vi "Autonomous Independent.vi"() -> ()   [LabVIEW 2014]
doc: "This VI is called when autonomous begins, and will automatically be terminated when autonomous ends. You can carry out timed or sensor driven robot movement independently without needing to return to the caller."
uses:
  <vilib>/Rock Robotics/WPI/Joystick/WPI_JoystickGetSetRefNum.vi
  Global Variables.vi
panel:
  out "Elapsed Time (s)":dbl
  out "Case":i32
  out "Array":dbl[][](array[numeric])
  # "Be sure to right-click and choose Data Operations>>Make Current Value default if you want to save the array values with the VI"
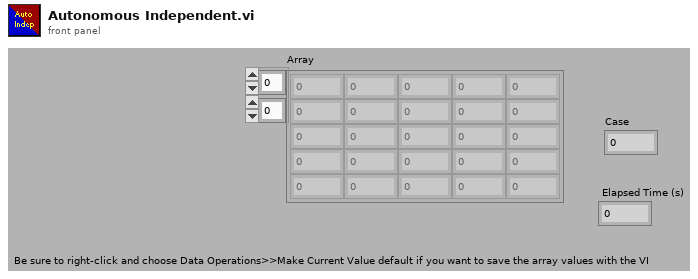
[diagram p1: front panel]
types:
  T1 = typedef "WPI_JoystickDevRef.ctl" = cluster{"Device":T2}
  T2 = typedef "WPI_JoystickDeviceEnum.ctl" = enum16{"USB 0", "USB 1", "USB 2", "USB 3", "USB 4", "USB 5"}
  T3 = typedef "WPI_CounterDevRef.ctl" = cluster{"DevStatus":errorcluster, "CntIndex":T4}
  T4 = typedef "FPGA_CounterCtrSystemIndex.ctl" = enum8{"Ctr 0", "Ctr 1", "Ctr 2", "Ctr 3", "Ctr 4", "Ctr 5", "Ctr 6", "Ctr 7", "Invalid"}
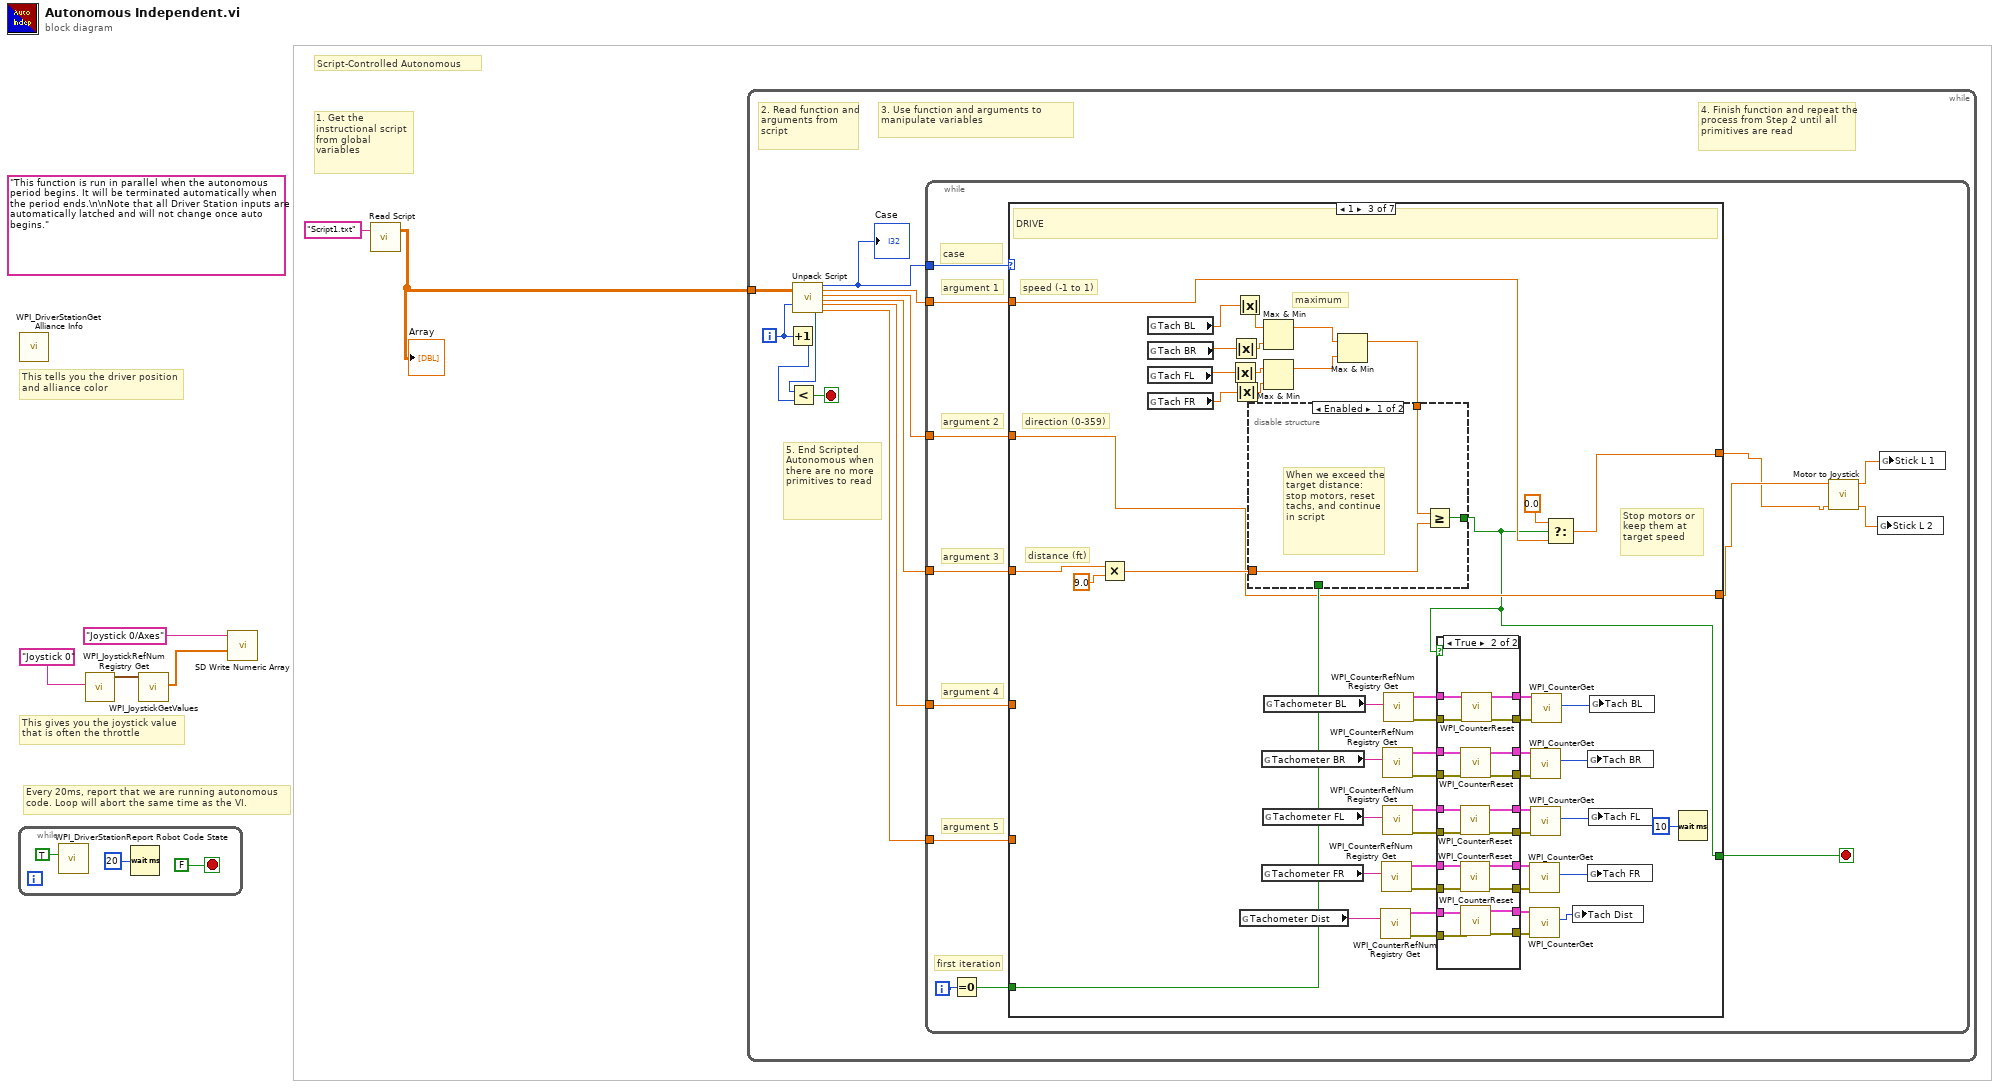
[diagram p0: block diagram]
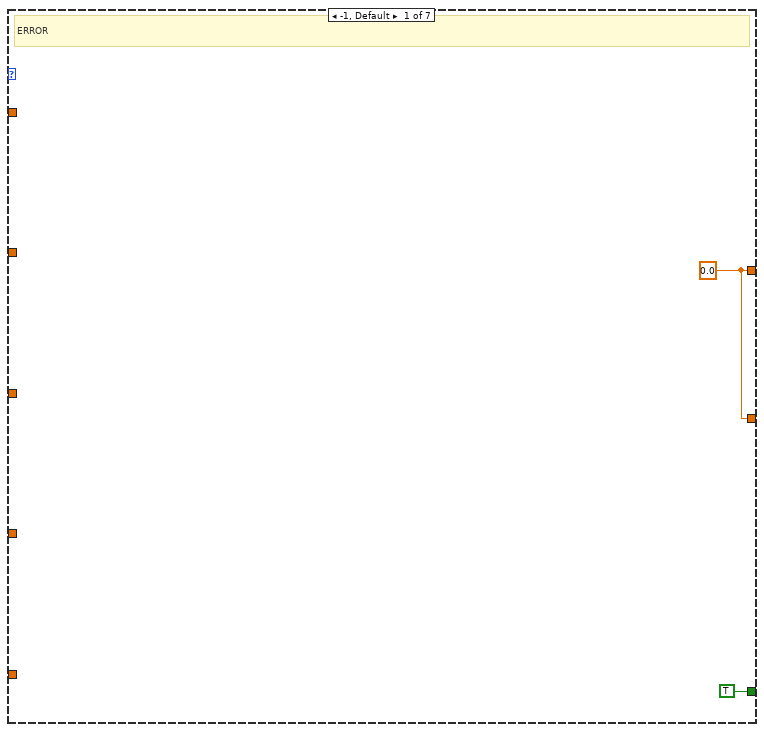
[diagram p2: hidden frame]
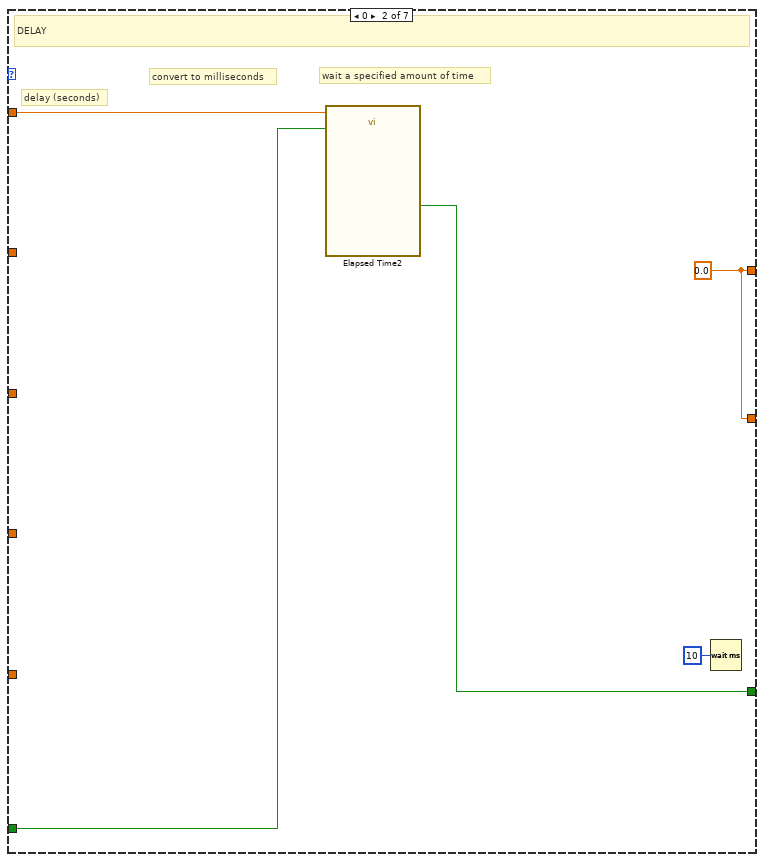
[diagram p3: hidden frame]
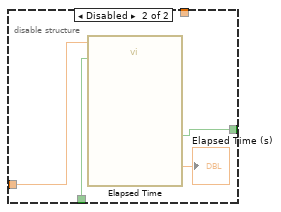
[diagram p5: hidden frame]
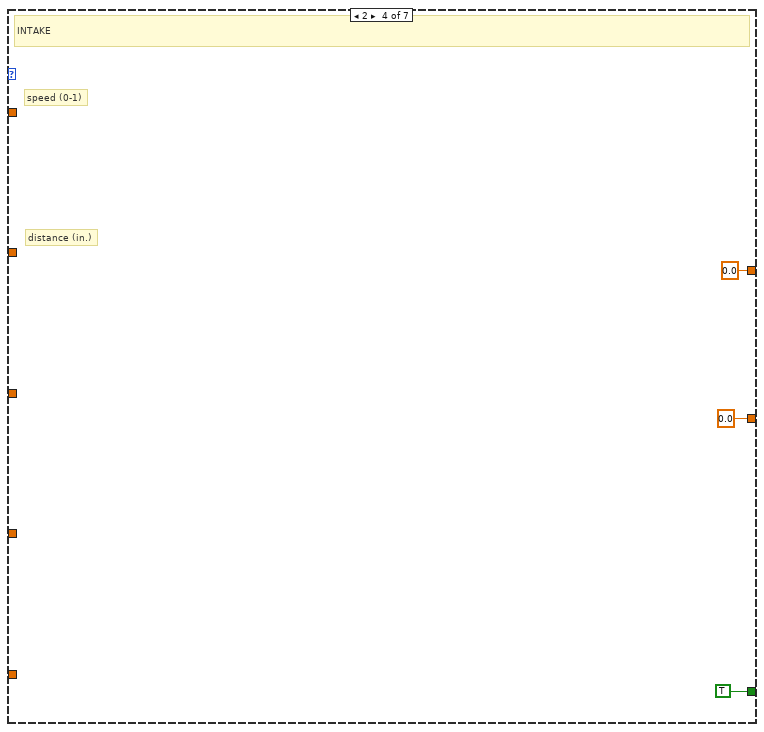
[diagram p6: hidden frame]
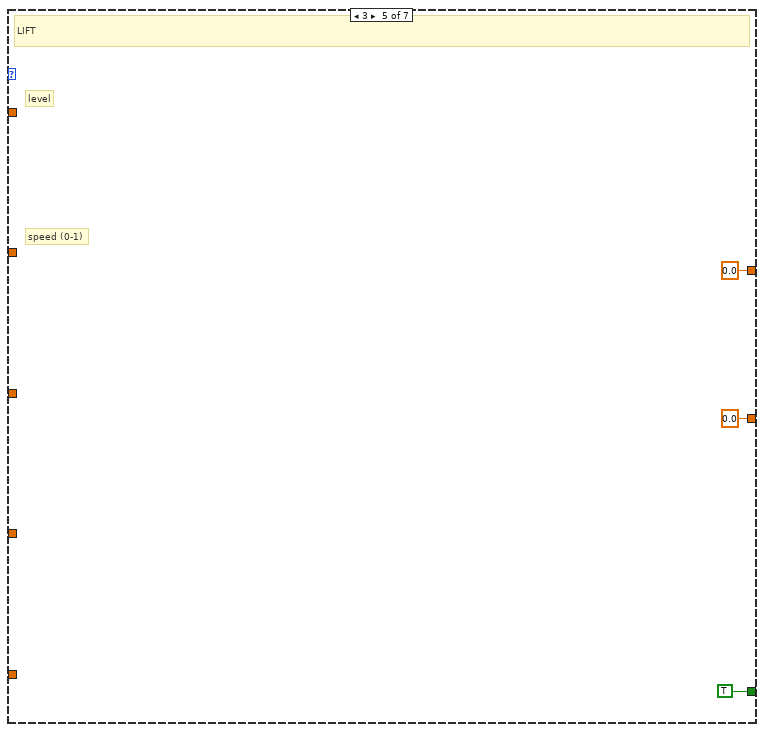
[diagram p7: hidden frame]
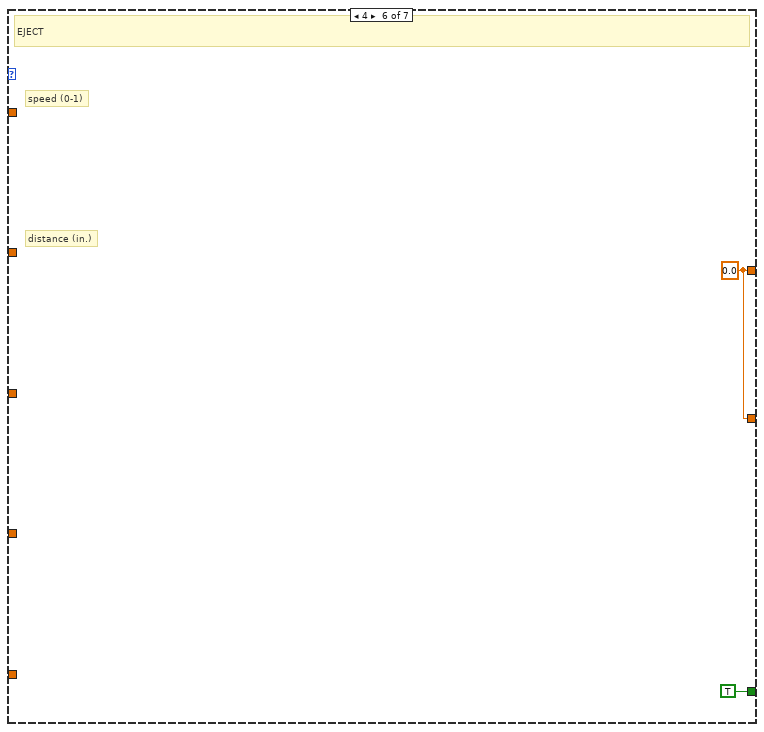
[diagram p8: hidden frame]
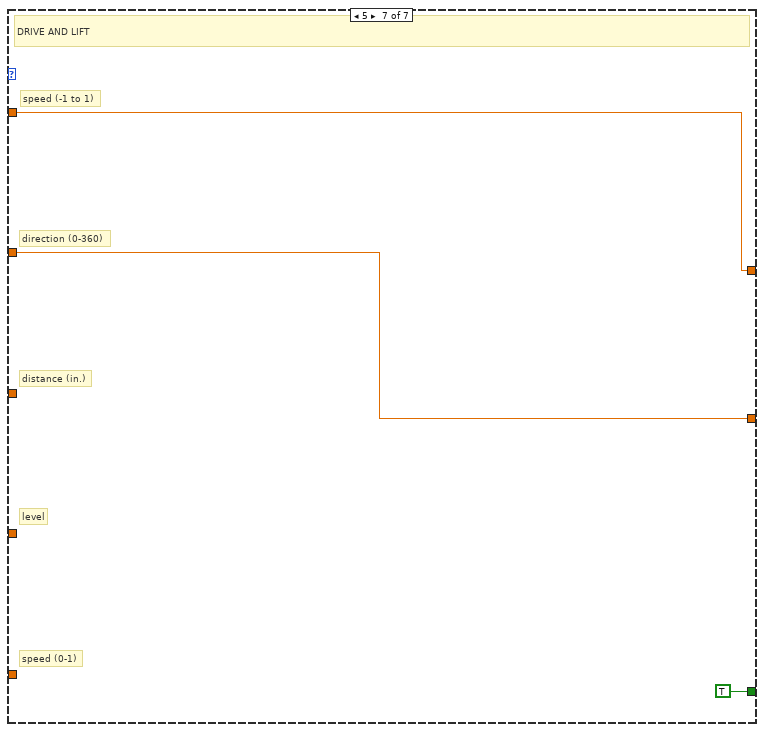
[diagram p9: hidden frame]
diagram:
  (unwired) "This function is run in parallel when the autonomous period begins. It will be terminated automatically when the period ends.\n\nNote that all Driver Station inputs are automatically latched and will not change once auto begins."
  # "1. Get the instructional script from global variables"
  # "Script-Controlled Autonomous"
  # "Every 20ms, report that we are running autonomous\ncode. Loop will abort the same time as the VI."
  # "This gives you the joystick value\nthat is often the throttle"
  # "This tells you the driver position\nand alliance color"
  n1 = while {
    stop <- FALSE stop-if-true
    n2 = call <vilib>:"WPI_DriverStationReport Robot Code State.vi"("Autonomous"=TRUE) -> ()  [unwired: 10 in, 1 out]
    n3 = Wait (ms)(milliseconds to wait=u32 20) -> ()  [unwired: 1 out]
  }
  n4 = call <vilib>:"WPI_DriverStationGet Alliance Info.vi"() -> ()  [unwired: 12 out]
  n5 = call <vilib>:"WPI_JoystickRefNum Registry Get.vi"("refnum name"="Joystick 0") -> ("JoystickDevRef"=w5:T1)  [unwired: 1 in, 9 out]
  n6 = call <vilib>:"WPI_JoystickGetValues.vi"("JoystickDevRef"=w5) -> ("Axes"=w3:dbl[])  [unwired: 6 in, 4 out]
  n7 = call <vilib>:"SD Write Numeric Array.vi"("Numeric Array"=w3, "Name"="Joystick 0/Axes") -> ()  [unwired: 8 in, 2 out]
  n8 = call "Read Script.vi"("script name"="Script1.txt") -> ("output array"=w1:dbl[][])  [unwired: 1 in, 1 out]
  "Array" <- w1
  n9 = while {
    tunnel: w1 -> [w11]
    i -> [w14]
    stop <- w20 stop-if-true
    # "4. Finish function and repeat the process from Step 2 until all primitives are read"
    # "3. Use function and arguments to manipulate variables"
    # "5. End Scripted Autonomous when there are no more primitives to read"
    # "2. Read function and arguments from script"
    n10 = Increment(x=w14) -> (x+1=w13:i32)
    n11 = call "Unpack Script.vi"("script"=w11, "index"=w14) -> ("# of primitives"=w12:i32, "primitive"=w10:i32, "argument 1"=w19:dbl, "argument 2"=w18:dbl, "argument 3"=w17:dbl, "argument 4"=w16:dbl, "argument 5"=w15:dbl)  [unwired: 11 in]
    "Case" <- w10
    n12 = Less?(x=w12, y=w13) -> (x < y?=w20:bool)
    n13 = while {
      tunnel: w19 -> [w33]
      tunnel: w18 -> [w32]
      tunnel: w17 -> [w31]
      tunnel: w16 -> [w30]
      tunnel: w15 -> [w29]
      tunnel: w10 -> [w28]
      i -> [w26]
      stop <- w27 stop-if-true
      # "first iteration"
      # "case"
      # "argument 5"
      # "argument 4"
      # "argument 3"
      # "argument 2"
      # "argument 1"
      n14 = Equal To 0?(x=w26) -> (x = 0?=w25:bool)
      n15 = case shown="1" w28 {
        tunnel: w33 -> [_ w40 w91 _ _ _ w138]
        tunnel: w32 -> [_ _ w80 _ _ _ w137]
        tunnel: w31 -> [_ _ w87 _ _ _ _]
        tunnel: w30 -> [_ _ _ _ _ _ _]
        tunnel: w29 -> [_ _ _ _ _ _ _]
        tunnel: [TRUE w38 w41 TRUE TRUE TRUE TRUE] -> w27
        tunnel: w25 -> [_ w39 w88 _ _ _ _]
        tunnel: [w34 w36 w81 0.0 ("argument 1") 0.0 ("argument 1") w135 w138] -> w23
        tunnel: [w34 w36 w80 0.0 ("argument 2") 0.0 ("argument 2") w135 w137] -> w24
        frame -1, Default {
          w34 = 0.0 ("argument 1")
          # "ERROR"
        }
        frame 0 {
          w36 = 0.0 ("argument 1")
          # "wait a specified amount of time"
          # "convert to milliseconds"
          # "delay (seconds)"
          # "DELAY"
          n16 = call "Elapsed Time2"("Time Target (s)"=w40, "Reset"=w39) -> ("Time has Elapsed"=w38:bool)  [unwired: 10 in, 7 out]
          n17 = Wait (ms)(milliseconds to wait=u32 10) -> ()  [unwired: 1 out]
        }
        frame 1 {
          # "maximum"
          # "Stop motors or keep them at target speed"
          # "distance (ft)"
          # "direction (0-359)"
          # "speed (-1 to 1)"
          # "DRIVE"
          n18 = Multiply(x=w87, y=9.0) -> (x*y=w85:dbl)
          n19 = global read "Global Variables.vi" "Tach BL"() -> (w73:dbl)
          n20 = global read "Global Variables.vi" "Tach BR"() -> (w74:dbl)
          n21 = global read "Global Variables.vi" "Tach FL"() -> (w75:dbl)
          n22 = global read "Global Variables.vi" "Tach FR"() -> (w76:dbl)
          n23 = Absolute Value(x=w75) -> (abs(x)=w78:dbl)
          n24 = Absolute Value(x=w74) -> (abs(x)=w79:dbl)
          n25 = Absolute Value(x=w76) -> (abs(x)=w77:dbl)
          n26 = Absolute Value(x=w73) -> (abs(x)=w72:dbl)
          n27 = global read "Global Variables.vi" "Tachometer Dist"() -> (w45:string)
          n28 = global read "Global Variables.vi" "Tachometer BR"() -> (w60:string)
          n29 = global read "Global Variables.vi" "Tachometer FR"() -> (w48:string)
          n30 = global read "Global Variables.vi" "Tachometer FL"() -> (w59:string)
          n31 = Max & Min(x=w72, y=w79) -> (max(x,y)=w84:dbl)  [unwired: 1 out]
          n32 = Max & Min(x=w78, y=w77) -> (max(x,y)=w83:dbl)  [unwired: 1 out]
          n33 = global read "Global Variables.vi" "Tachometer BL"() -> (w71:string)
          n34 = Max & Min(x=w84, y=w83) -> (max(x,y)=w82:dbl)  [unwired: 1 out]
          n35 = disable-structure shown="Enabled" {
            disable-tunnel: w85 -> [w124 w126]
            disable-tunnel: [w123 w128] -> w41
            disable-tunnel: w88 -> [_ w125]
            disable-tunnel: w82 -> [w122 _]
            frame Enabled {
              # "When we exceed the target distance: stop motors, reset tachs, and continue in script"
              n36 = Greater Or Equal?(x=w122, y=w124) -> (x >= y?=w123:bool)
            }
            frame Disabled {
              n37 = call "Elapsed Time"("Time Target (s)"=w126, "Reset"=w125) -> ("Elapsed Time (s)"=→"Elapsed Time (s)":dbl, "Time has Elapsed"=w128:bool)  [unwired: 10 in, 6 out]
            }
          }
          n38 = call <vilib>:"WPI_CounterRefNum Registry Get.vi"("refnum name"=w45) -> ("error out"=w43:errorcluster, "CounterDevRef"=w47:T3)  [unwired: 9 in]
          n39 = call <vilib>:"WPI_CounterRefNum Registry Get.vi"("refnum name"=w48) -> ("error out"=w50:errorcluster, "CounterDevRef"=w49:T3)  [unwired: 9 in]
          n40 = call <vilib>:"WPI_CounterRefNum Registry Get.vi"("refnum name"=w60) -> ("error out"=w62:errorcluster, "CounterDevRef"=w61:T3)  [unwired: 9 in]
          n41 = call <vilib>:"WPI_CounterRefNum Registry Get.vi"("refnum name"=w59) -> ("error out"=w57:errorcluster, "CounterDevRef"=w58:T3)  [unwired: 9 in]
          n42 = call <vilib>:"WPI_CounterRefNum Registry Get.vi"("refnum name"=w71) -> ("error out"=w69:errorcluster, "CounterDevRef"=w70:T3)  [unwired: 9 in]
          n43 = case shown="True" w41 {
            tunnel: w70 -> [w101 w121]
            tunnel: w69 -> [w100 w120]
            tunnel: [w101 w119] -> w68
            tunnel: [w100 w118] -> w67
            tunnel: w61 -> [w98 w108]
            tunnel: w62 -> [w99 w117]
            tunnel: [w98 w107] -> w63
            tunnel: [w99 w106] -> w64
            tunnel: w58 -> [w97 w109]
            tunnel: w57 -> [w96 w116]
            tunnel: [w97 w110] -> w56
            tunnel: [w96 w111] -> w55
            tunnel: w49 -> [w94 w114]
            tunnel: w50 -> [w95 w115]
            tunnel: [w94 w113] -> w51
            tunnel: [w95 w112] -> w52
            tunnel: w47 -> [w93 w105]
            tunnel: [w93 w104] -> w46
            tunnel: w43 -> [w92 w103]
            tunnel: [w92 w102] -> w42
            frame False {
            }
            frame True {
              n44 = call <vilib>:"WPI_CounterReset.vi"("error in (no error)"=w116, "CounterDevRef in"=w109) -> ("error out"=w111:errorcluster, "CounterDevRef out"=w110:T3)  [unwired: 8 in]
              n45 = call <vilib>:"WPI_CounterReset.vi"("error in (no error)"=w115, "CounterDevRef in"=w114) -> ("error out"=w112:errorcluster, "CounterDevRef out"=w113:T3)  [unwired: 8 in]
              n46 = call <vilib>:"WPI_CounterReset.vi"("error in (no error)"=w117, "CounterDevRef in"=w108) -> ("error out"=w106:errorcluster, "CounterDevRef out"=w107:T3)  [unwired: 8 in]
              n47 = call <vilib>:"WPI_CounterReset.vi"("error in (no error)"=w103, "CounterDevRef in"=w105) -> ("error out"=w102:errorcluster, "CounterDevRef out"=w104:T3)  [unwired: 8 in]
              n48 = call <vilib>:"WPI_CounterReset.vi"("error in (no error)"=w120, "CounterDevRef in"=w121) -> ("error out"=w118:errorcluster, "CounterDevRef out"=w119:T3)  [unwired: 8 in]
            }
          }
          n49 = call <vilib>:"WPI_CounterGet.vi"("error in (no error)"=w52, "CounterDevRef in"=w51) -> ("Value"=w53:i32)  [unwired: 4 in, 5 out]
          n50 = call <vilib>:"WPI_CounterGet.vi"("error in (no error)"=w42, "CounterDevRef in"=w46) -> ("Value"=w44:i32)  [unwired: 4 in, 5 out]
          n51 = call <vilib>:"WPI_CounterGet.vi"("error in (no error)"=w64, "CounterDevRef in"=w63) -> ("Value"=w65:i32)  [unwired: 4 in, 5 out]
          n52 = call <vilib>:"WPI_CounterGet.vi"("error in (no error)"=w55, "CounterDevRef in"=w56) -> ("Value"=w54:i32)  [unwired: 4 in, 5 out]
          n53 = call <vilib>:"WPI_CounterGet.vi"("error in (no error)"=w67, "CounterDevRef in"=w68) -> ("Value"=w66:i32)  [unwired: 4 in, 5 out]
          n54 = Select(t=0.0, s=w41, f=w91) -> (s? t:f=w81:dbl)
          n55 = global write "Global Variables.vi" "Tach Dist"(w44) -> ()
          n56 = global write "Global Variables.vi" "Tach BR"(w65) -> ()
          n57 = global write "Global Variables.vi" "Tach FR"(w53) -> ()
          n58 = global write "Global Variables.vi" "Tach FL"(w54) -> ()
          n59 = global write "Global Variables.vi" "Tach BL"(w66) -> ()
          n60 = Wait (ms)(milliseconds to wait=u32 10) -> ()  [unwired: 1 out]
        }
        frame 2 {
          # "distance (in.)"
          # "speed (0-1)"
          # "INTAKE"
        }
        frame 3 {
          # "speed (0-1)"
          # "level"
          # "LIFT"
        }
        frame 4 {
          w135 = 0.0 ("argument 1")
          # "distance (in.)"
          # "speed (0-1)"
          # "EJECT"
        }
        frame 5 {
          # "speed (0-1)"
          # "level"
          # "distance (in.)"
          # "direction (0-360)"
          # "speed (-1 to 1)"
          # "DRIVE AND LIFT"
        }
      }
      n61 = call "Motor to Joystick.vi"("Drive Motor"=w23, "Rotational Motor"=w24) -> ("Joy Y"=w21:dbl, "Joy X"=w22:dbl)  [unwired: 8 in]
      n62 = global write "Global Variables.vi" "Stick L 2"(w21) -> ()
      n63 = global write "Global Variables.vi" "Stick L 1"(w22) -> ()
    }
  }
